vi "Server Create Response Event.vi"(8 "error in":errorcluster, 11 "server ref":refnum<vi>) -> (0 "error out":errorcluster, 3 "user event out":T1)   [LabVIEW 2020]
doc: "Create user event for server operation answers. I.e.: for sending query command answer from TWM to server."
uses:
  Server Event Answer Ref.ctl
  Server Session Reference.ctl
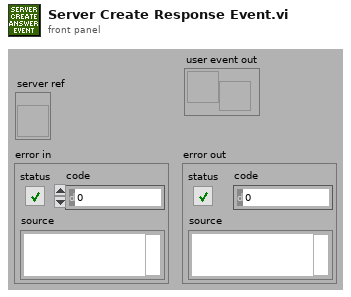
[diagram p1: front panel]
types:
  T1 = typedef "Server Event Answer Ref.ctl" = refnum<user-event>
  T2 = typedef "Server Session Reference.ctl" = refnum<vi>
  T3 = typedef "Server Session.ctl" = cluster{"cmd event":variant, "answer event":variant}
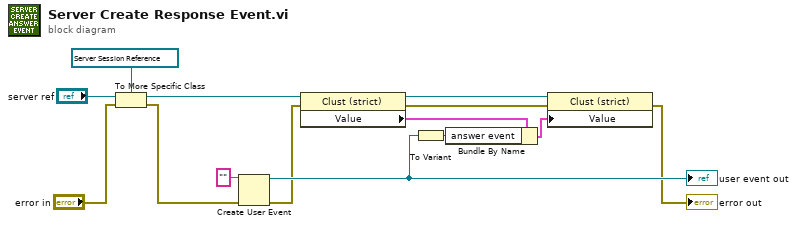
[diagram p0: block diagram]
diagram:
  n1 = To More Specific Class(target class=T2 refnum ("server ref"), reference="server ref", error in="error in") -> (specific class reference=w8:T2, error out=w10:errorcluster)
  n2 = Create User Event(user event datatype="" ("String"), error in=w10) -> (user event=w14:refnum<user-event>, error out=w6:errorcluster)
  "user event out" <- w14
  n3 = property class="Clust (strict)"(reference=w8, error in=w6) -> (reference out=w7:T2, error out=w5:errorcluster, "Value"=w4:T3)
  n4 = To Variant(anything=w14) -> (Variant=w2:variant)
  n5 = Bundle By Name(cluster=w4, "answer event"=w2) -> (w3:T3)
  n6 = property class="Clust (strict)"(reference=w7, error in=w5, "Value"=w3) -> (error out=→"error out":errorcluster)  [unwired: 1 out]
